vi "Mouse Down on Marker MinMax.vi"(8 "error in (no error)":errorcluster, 11 "Scale ref":refnum<vi>) -> (0 "error out":errorcluster, 2 "mouse down on marker min/max?":bool, 3 "scale ref":refnum<vi>)   [LabVIEW 2021, in "RocketPlot.lvlib"]
uses:
  RocketPlot.lvlib
  <vilib>/Utility/miscctls.llb/LVSelectionTypeDef.ctl
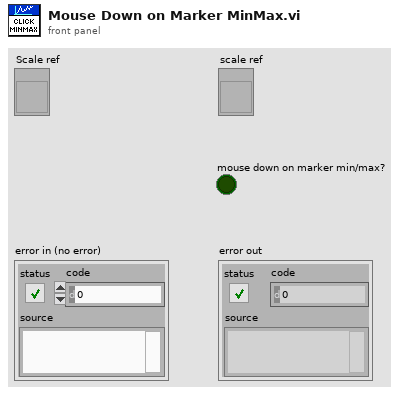
[diagram p1: front panel]
types:
  T1 = typedef "LVRangeTypeDef.ctl" = cluster{"Minimum":dbl, "Maximum":dbl, "Increment":dbl, "Minor Increment":dbl, "Start":dbl}
  T2 = typedef "LVSelectionTypeDef.ctl" = cluster{"Selection Start":u32, "Selection End":u32}
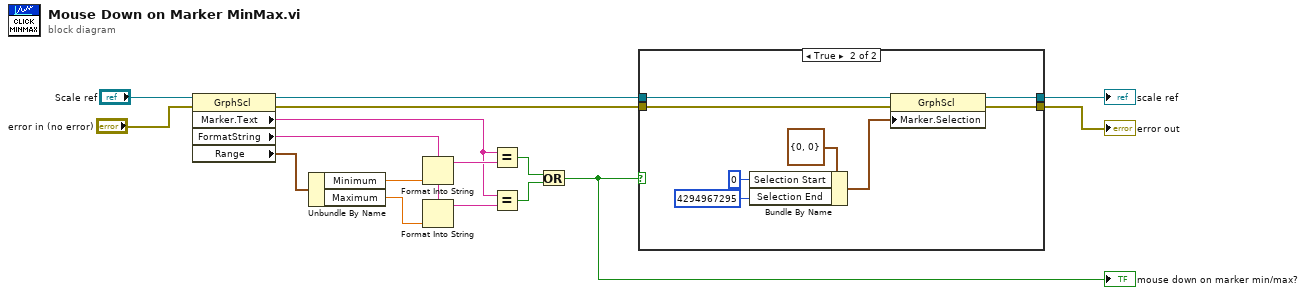
[diagram p0: block diagram]
diagram:
  n1 = property class="GrphScl"(reference="Scale ref", error in="error in (no error)") -> (reference out=w5:refnum<vi>, error out=w2:errorcluster, "Marker.Text"=w9:string, "FormatString"=w12:string, "Range"=w15:T1)
  n2 = Unbundle By Name(w15) -> ("Minimum"=w14:dbl, "Maximum"=w13:dbl)
  n3 = Format Into String(format string=w12, w14) -> (resulting string=w11:string)  [unwired: 2 in, 1 out]
  n4 = Format Into String(format string=w12, w13) -> (resulting string=w10:string)  [unwired: 2 in, 1 out]
  n5 = Equal?(x=w9, y=w11) -> (x = y?=w8:bool)
  n6 = Equal?(x=w9, y=w10) -> (x = y?=w7:bool)
  n7 = Or(x=w8, y=w7) -> (x .or. y?=w4:bool)
  "mouse down on marker min/max?" <- w4
  n8 = case shown="True" w4 {
    tunnel: w5 -> [w18 w22]
    tunnel: [w18 w21] -> w3
    tunnel: w2 -> [w17 w20]
    tunnel: [w17 w19] -> w1
    frame False {
    }
    frame True {
      n9 = Bundle By Name(cluster=T2 {"Selection Start"=0, "Selection End"=0} ("Marker.Selection"), "Selection Start"=u32 0, "Selection End"=u32 4294967295) -> (w23:T2)
      n10 = property class="GrphScl"(reference=w22, error in=w20, "Marker.Selection"=w23) -> (reference out=w21:refnum<vi>, error out=w19:errorcluster)
    }
  }
  "error out" <- w1
  "scale ref" <- w3
